vi "Read_Real_Speed_Command.vi"() -> (0 "Read Real Speed String to send:":string)   [LabVIEW 2019]
doc: "This vi sends to inverter a command to read the real speed.\nIt can be used anytime in both serial or drop-in control speed.\nSometimes, real speed could be different of sent speed because of load conditions."
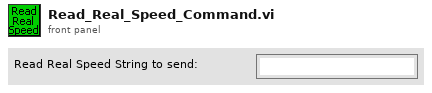
[diagram p1: front panel]
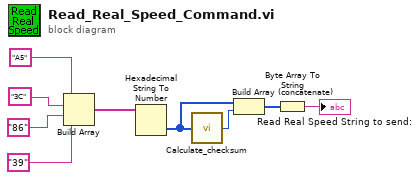
[diagram p0: block diagram]
diagram:
  n1 = Build Array("A5", "3C", "86", "39") -> (w4:string[])
  n2 = Hexadecimal String To Number(string=w4) -> (number=w2:u32[])  [unwired: 2 in, 1 out]
  n3 = call "Calculate_checksum.vi"("Data"=w2) -> ("Checksum"=w3:i32)
  n4 = Build Array (concatenate)(w2, w3) -> (w5:u32[])
  n5 = Byte Array To String(unsigned byte array=w5) -> (string=→"Read Real Speed String to send:":string)
